vi "RT Microprocessor.vi"() -> ()   [LabVIEW 2015]
doc: "This is the primary Real-Time VI."
uses:
  <vilib>/EmbeddedDisplay/Hitachi HD44780/Common/Control/screen size.ctl
  <vilib>/EmbeddedDisplay/Hitachi HD44780/Common/Control/font configuration.ctl
  <vilib>/EmbeddedDisplay/Hitachi HD44780/Common/Control/cursor position.ctl
  <vilib>/FPGAPlugInAG/sbRIO-9636/niLvFpga_Open_sbRIO-9636.vi
  <vilib>/rvi/interface/common/dynamic/niFpgaDynamicAddResources.vi
  <vilib>/FPGAPlugInAG/Dynamic/niLvFpga_Reset_Dynamic.vi
  <vilib>/FPGAPlugInAG/Dynamic/niLvFpga_Run_Dynamic.vi
  <vilib>/Utility/error.llb/Error Cluster From Error Code.vi
  <vilib>/rvi/errors/niLvFpgaAdjustHostInterfaceError.vi
  <vilib>/EmbeddedDisplay/Hitachi HD44780/Host/Public/Output (String).vi
  <vilib>/FPGAPlugInAG/Dynamic/niLvFpga_Close_Dynamic.vi
  <vilib>/rvi/interface/nirviOpenFPGA/nirviOpenFPGA.xnode
  2-_Create_FPGA_Application/2- Create FPGA Application/FPGA Bitfiles/Exercise2_FPGATarget_Exercise2_131A8AF0.lvbitx
  <vilib>/rvi/interface/nirviMethod/nirviMethod.xnode
  <vilib>/rvi/interface/nirviReadWriteControl/nirviReadWriteControl.xnode
  <vilib>/rvi/interface/nirviCloseFPGA/nirviCloseFPGA.xnode
  NiFpgaLv.dll
  <vilib>/rvi/interface/Simulation/niFpgaSimulationCallBeginRW.vi
  <vilib>/EmbeddedDisplay/Hitachi HD44780/Host/HD44780 Host.lvlib
  <vilib>/EmbeddedDisplay/Hitachi HD44780/Common/HD44780 Common.lvlib
panel:
  in  "Max Temp":fxp<+/-,32,13>=33.0
  out "RPM":fxp<+,32,16>
  out "Temp":fxp<+/-,32,13>
  out "Voltage":fxp<+/-,24,5>
  out "Battery State":enum16{"Charged", "Running", "Low Batt"}(ring)
  out "Temp Warning":bool
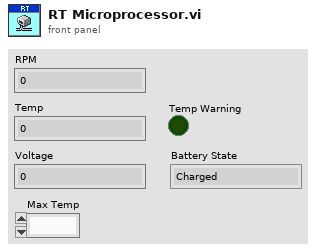
[diagram p1: front panel]
types:
  T1 = typedef "HD44780 Common.lvlib/font configuration.ctl" = enum8{"5x8 & 2 lines", "5x10 & 1 line", "5x8 & 1 line"}
  T2 = typedef "HD44780 Common.lvlib/screen size.ctl" = enum8{"8x1", "8x2", "12x4", "16x1", "16x2", "16x4", "20x1", "20x2", "20x4", "24x1", "24x2", "40x2", "40x4"}
  T3 = typedef "HD44780 Common.lvlib/cursor position.ctl" = cluster{"row":i8, "column":i8}
  T4 = enum16{"Battery State", "RPM", "Temp", "Voltage"}
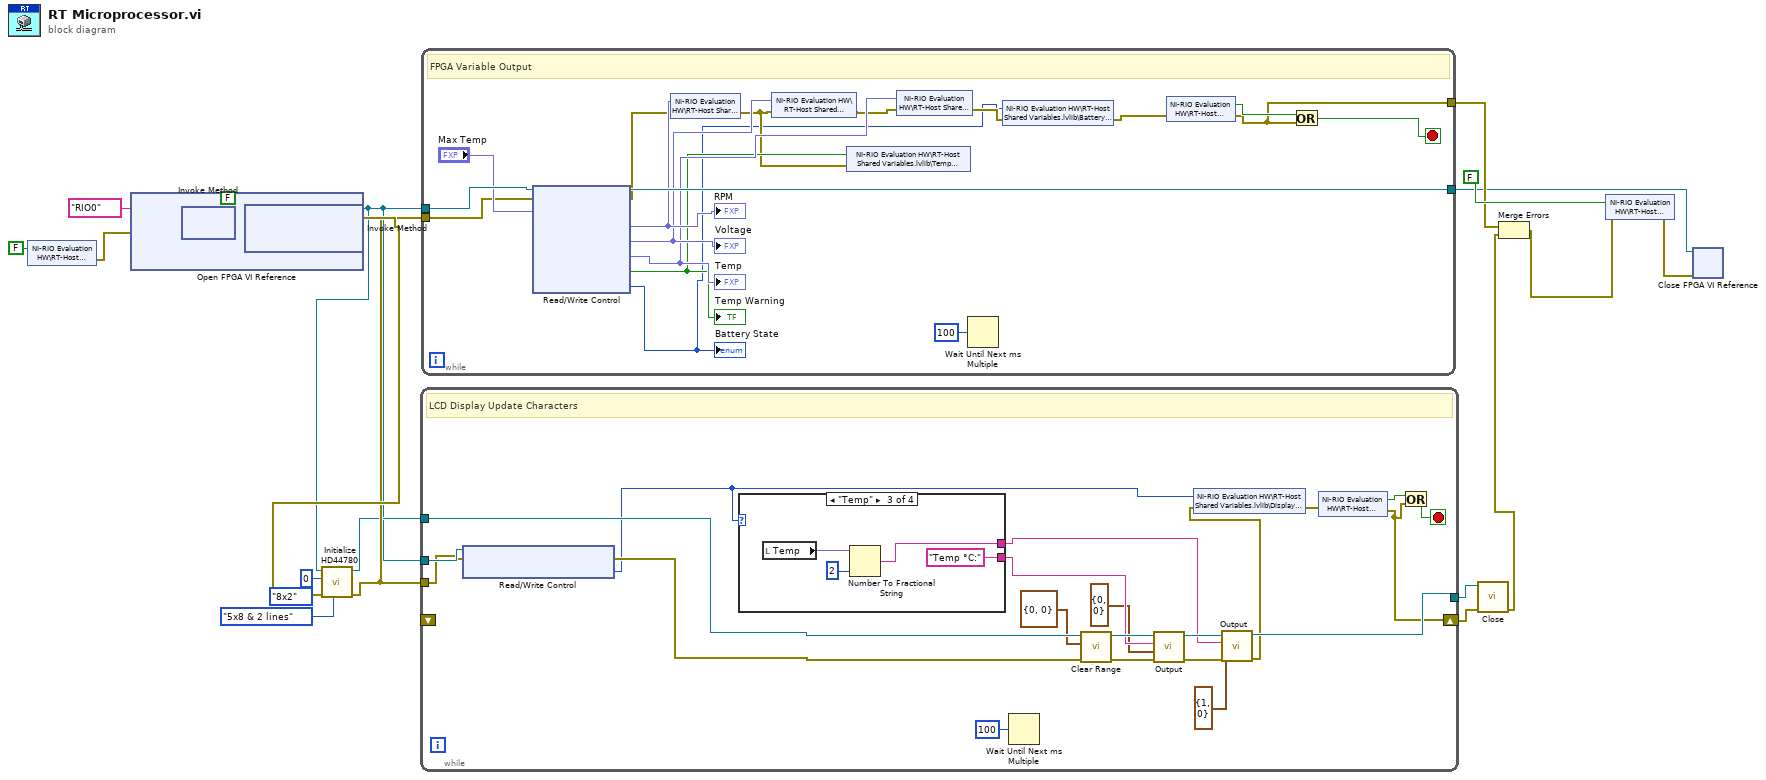
[diagram p0: block diagram]
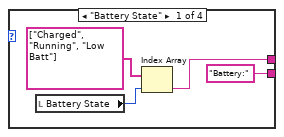
[diagram p2: hidden frame]
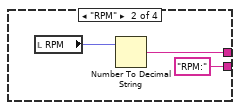
[diagram p3: hidden frame]
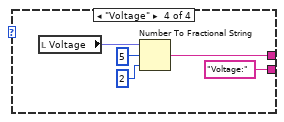
[diagram p4: hidden frame]
diagram:
  n1 = shared-variable "NI-RIO Evaluation HW\\RT-Host Shared Variables.lvlib\\Stop"(FALSE ("Stop")) -> (error out=w13:errorcluster)  [unwired: 1 in]
  n2 = xnode "Open FPGA VI Reference"("error in"=w13, "resource name"=tag "RIO0") -> ("FPGA VI Reference Out"=w23:refnum<k20>, "error out"=w12:errorcluster)
  n3 = xnode "Invoke Method"("FPGA VI Reference In"=w23, "error in"=w12) -> ("FPGA VI Reference Out"=w22:refnum<k20>, "error out"=w11:errorcluster)
  n4 = xnode "Invoke Method"("FPGA VI Reference In"=w22, "error in"=w11, "Wait Until Done (F)"=FALSE) -> ("FPGA VI Reference Out"=w2:refnum<k20>, "error out"=w21:errorcluster)
  n5 = call <vilib>:"Initialize HD44780.vi"("font configuration (5x8 & 2 lines)"=font_configuration."5x8 & 2 lines", "error in (no error)"=w21, "screen size"=screen_size."8x2", "device index"=i8 0, "FPGA VI Reference in"=w2) -> ("error out"=w20:errorcluster, "LCD out"=w16:refnum<class "Character LCD.lvclass">)  [unwired: 5 in]
  n6 = while {
    tunnel: w2 -> [w44]
    tunnel: w20 -> [w43]
    tunnel: w16 -> [w39]
    tunnel: [w36] -> w15
    shift-right: [w27] -> w6
    shift-left: _ -> [_]
    stop <- w29 stop-if-true
    # "LCD Display Update Characters"
    n7 = xnode "Read/Write Control"("FPGA VI Reference In"=w44, "error in"=w43) -> ("error out"=w42:errorcluster, "FPGA Display Command"=w25:T4)  [unwired: 1 out]
    n8 = case shown="\"Temp\"" w25 {
      tunnel: ["Battery:" "RPM:" "Temp °C:" "Voltage:"] -> w35
      tunnel: [w47 w50 w53 w58] -> w34
      frame "Battery State" {
        n9 = local read "Battery State"() -> (w46:enum16{"Charged", "Running", "Low Batt"})
        n10 = Index Array(array=string[] ["Charged", "Running", "Low Batt"], index=w46) -> (element=w47:string)
      }
      frame "RPM" {
        n11 = local read "RPM"() -> (w49:fxp<+,32,16>)
        n12 = Number To Decimal String(number=w49) -> (decimal integer string=w50:string)  [unwired: 1 in]
      }
      frame "Temp" {
        n13 = local read "Temp"() -> (w52:fxp<+/-,32,13>)
        n14 = Number To Fractional String(number=w52, precision (6)=i16 2) -> (F-format string=w53:string)  [unwired: 2 in]
      }
      frame "Voltage" {
        n15 = local read "Voltage"() -> (w56:fxp<+/-,24,5>)
        n16 = Number To Fractional String(number=w56, width (-)=i16 5, precision (6)=i16 2) -> (F-format string=w58:string)  [unwired: 1 in]
      }
    }
    n17 = Wait Until Next ms Multiple(millisecond multiple=u32 100) -> ()  [unwired: 1 out]
    n18 = call <vilib>:"Clear Range.vi"("error in (no error)"=w42, "start position"=T3 {"row"=0, "column"=0}, "LCD in"=w39) -> ("error out"=w41:errorcluster, "LCD out"=w38:refnum<class "Character LCD.lvclass">)  [unwired: 7 in]
    n19 = call-poly <vilib>:"Output.vi"("error in (no error)"=w41, "position"=T3 {"row"=0, "column"=0}, "text"=w35, "LCD in"=w38) -> ("error out"=w40:errorcluster, "LCD out"=w37:refnum<class "Character LCD.lvclass">)  [unwired: 5 in, 1 out]
    n20 = call-poly <vilib>:"Output.vi"("error in (no error)"=w40, "position"=T3 {"row"=1, "column"=0}, "text"=w34, "LCD in"=w37) -> ("error out"=w31:errorcluster, "LCD out"=w36:refnum<class "Character LCD.lvclass">)  [unwired: 5 in, 1 out]
    n21 = shared-variable "NI-RIO Evaluation HW\\RT-Host Shared Variables.lvlib\\Display State"(w25, error in=w31) -> (error out=w30:errorcluster)
    n22 = shared-variable "NI-RIO Evaluation HW\\RT-Host Shared Variables.lvlib\\Stop"(error in=w30) -> (w28:bool, error out=w27:errorcluster)
    n23 = Or(x=w28, y=w27) -> (x .or. y?=w29:bool)
  }
  n24 = while {
    tunnel: w2 -> [w78]
    tunnel: [w76] -> w4
    tunnel: [w64] -> w8
    tunnel: w20 -> [w62]
    stop <- w63 stop-if-true
    # "FPGA Variable Output"
    n25 = xnode "Read/Write Control"("FPGA VI Reference In"=w78, "error in"=w62, "Max Temp"="Max Temp") -> ("FPGA VI Reference Out"=w76:refnum<k20>, "error out"=w74:errorcluster, "RPM"=w75:fxp<+,32,16>, "Voltage"=w73:fxp<+/-,24,5>, "Temp"=w72:fxp<+/-,32,13>, "Temp Warning"=w70:bool, "Battery State"=w67:enum16{"Charged", "Running", "Low Batt"})
    "Temp Warning" <- w70
    "Battery State" <- w67
    "Voltage" <- w73
    "Temp" <- w72
    "RPM" <- w75
    n26 = shared-variable "NI-RIO Evaluation HW\\RT-Host Shared Variables.lvlib\\RPM"(w75, error in=w74) -> (error out=w69:errorcluster)
    n27 = shared-variable "NI-RIO Evaluation HW\\RT-Host Shared Variables.lvlib\\Voltage"(w73, error in=w69) -> (error out=w71:errorcluster)
    n28 = shared-variable "NI-RIO Evaluation HW\\RT-Host Shared Variables.lvlib\\Temp Warning"(w70, error in=w69) -> ()  [unwired: 1 out]
    n29 = shared-variable "NI-RIO Evaluation HW\\RT-Host Shared Variables.lvlib\\Temp"(w72, error in=w71) -> (error out=w68:errorcluster)
    n30 = Wait Until Next ms Multiple(millisecond multiple=u32 100) -> ()  [unwired: 1 out]
    n31 = shared-variable "NI-RIO Evaluation HW\\RT-Host Shared Variables.lvlib\\Battery State"(w67, error in=w68) -> (error out=w66:errorcluster)
    n32 = shared-variable "NI-RIO Evaluation HW\\RT-Host Shared Variables.lvlib\\Stop"(error in=w66) -> (w65:bool, error out=w64:errorcluster)
    n33 = Or(x=w65, y=w64) -> (x .or. y?=w63:bool)
  }
  n34 = call <vilib>:"Close.vi"("error in (no error)"=w6, "LCD in"=w15) -> ("error out"=w5:errorcluster)  [unwired: 9 in]
  n35 = Merge Errors(w8, w5) -> (w7:errorcluster)
  n36 = shared-variable "NI-RIO Evaluation HW\\RT-Host Shared Variables.lvlib\\Stop"(FALSE ("Stop"), error in=w7) -> (error out=w10:errorcluster)
  n37 = xnode "Close FPGA VI Reference"("FPGA VI Reference In"=w4, "error in"=w10) -> ()  [unwired: 1 out]
